vi "Status.vi"(8 "error in (no error)":errorcluster, 11 "Huber Settings":T1) -> (0 "error out":errorcluster, 1 "Connection Error":bool, 2 "Running":bool, 3 "Huber Settings":T1, 4 "Temp":i32)   [LabVIEW 2018, in "Huber Ministat 230 TCU.lvlib"]
uses:
  Huber Ministat 230 TCU.lvlib
  Huber Settings.ctl
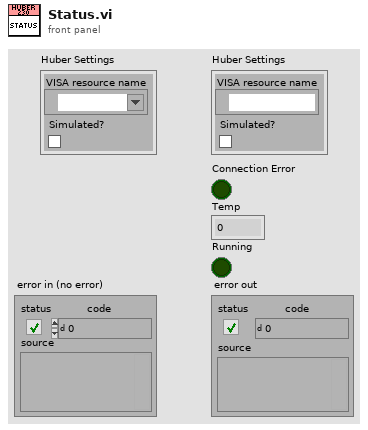
[diagram p1: front panel]
types:
  T1 = typedef "Huber Ministat 230 TCU.lvlib/Huber Settings.ctl" = cluster{"VISA resource name":refnum<visa-resource-name>, "Simulated?":bool}
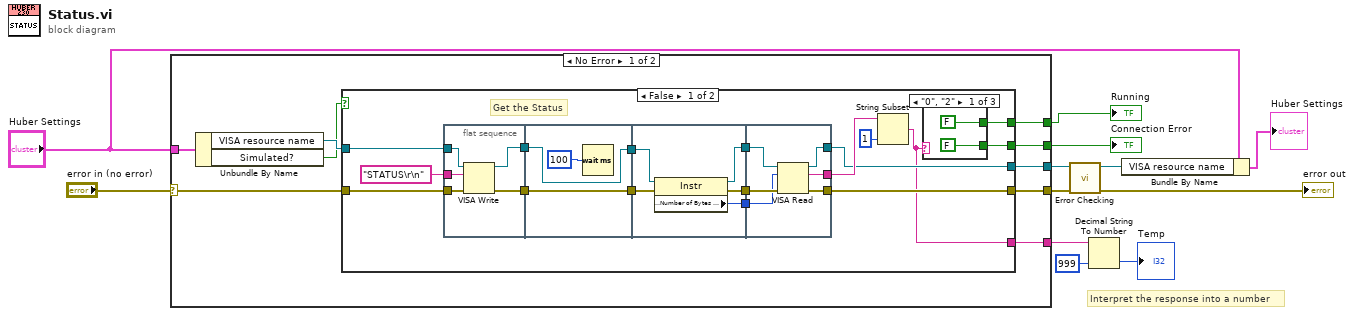
[diagram p0: block diagram]
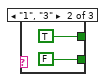
[diagram p2: hidden frame]
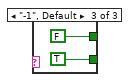
[diagram p3: hidden frame]
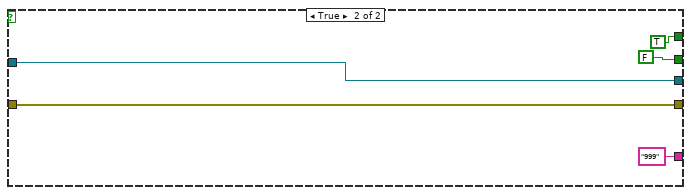
[diagram p4: hidden frame]
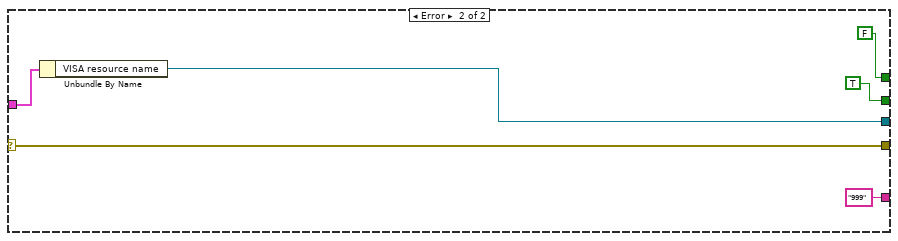
[diagram p5: hidden frame]
diagram:
  # "Interpret the response into a number"
  n1 = case shown="No Error" "error in (no error)" {
    selector: "error in (no error)" -> [w21 w74]
    tunnel: "Huber Settings" -> [w19 w73]
    tunnel: [w20 w74] -> w10
    tunnel: [w17 w72] -> w11
    tunnel: [w15 TRUE] -> w5
    tunnel: [w14 FALSE] -> w4
    tunnel: [w13 "999" ("read buffer")] -> w2
    frame No Error {
      n2 = Unbundle By Name(w19) -> ("VISA resource name"=w18:refnum<visa-resource-name>, "Simulated?"=w16:bool)
      n3 = case shown="False" w16 {
        tunnel: w21 -> [w24 w68]
        tunnel: [w26 w68] -> w20
        tunnel: [w27 w67] -> w17
        tunnel: w18 -> [w25 w67]
        tunnel: [w35 FALSE] -> w15
        tunnel: [w23 TRUE] -> w14
        tunnel: [w22 "999" ("read buffer")] -> w13
        frame False {
          # "Get the Status"
          n4 = flat-sequence {
            tunnel: "STATUS\r\n" ("string") -> [w49]
            tunnel: [w48] -> w37
            tunnel: [w47] -> w36
            tunnel: w25 -> [w46]
            tunnel: w24 -> [w45]
            tunnel: w37 -> [w51]
            tunnel: w36 -> [w50]
            tunnel: [w51] -> w29
            tunnel: [w50] -> w28
            tunnel: [w55] -> w32
            tunnel: [w54] -> w31
            tunnel: [w53] -> w30
            tunnel: w29 -> [w57]
            tunnel: w28 -> [w56]
            tunnel: [w63] -> w26
            tunnel: [w62] -> w33
            tunnel: [w61] -> w27
            tunnel: w32 -> [w60]
            tunnel: w31 -> [w59]
            tunnel: w30 -> [w58]
            frame #0 {
              n5 = VISA Write(VISA resource name=w46, write buffer=w49, error in (no error)=w45) -> (VISA resource name out=w48:refnum<visa-resource-name>, error out=w47:errorcluster)  [unwired: 1 out]
            }
            frame #1 {
              n6 = Wait (ms)(milliseconds to wait=u32 100) -> ()  [unwired: 1 out]
            }
            frame #2 {
              n7 = property class="Instr"(reference=w57, error in=w56) -> (reference out=w55:refnum<visa-resource-name>, error out=w54:errorcluster, "Serial Settings:Number of Bytes at Serial Port"=w53:u32)
            }
            frame #3 {
              n8 = VISA Read(VISA resource name=w60, byte count=w58, error in (no error)=w59) -> (VISA resource name out=w61:refnum<visa-resource-name>, read buffer=w62:string, error out=w63:errorcluster)  [unwired: 1 out]
            }
          }
          n9 = String Subset(string=w33, length (rest)=1 ("length (rest)")) -> (substring=w22:string)  [unwired: 1 in]
          n10 = case shown="\"0\", \"2\"" w22 {
            tunnel: [FALSE FALSE TRUE] -> w35
            tunnel: [FALSE TRUE FALSE] -> w23
            frame "0", "2" {
            }
            frame "1", "3" {
            }
            frame "-1", Default {
            }
          }
        }
        frame True {
        }
      }
    }
    frame Error {
      n11 = Unbundle By Name(w73) -> ("VISA resource name"=w72:refnum<visa-resource-name>)
    }
  }
  "Connection Error" <- w5
  "Running" <- w4
  n12 = call "Error Checking.vi"("error in (no error)"=w10, "VISA resource name"=w11) -> ("error out"=→"error out":errorcluster, "VISA resource name"=w8:refnum<visa-resource-name>)  [unwired: 7 in, 1 out]
  n13 = Decimal String To Number(string=w2, default (0L)=999 ("default (0 I32)")) -> (number=→"Temp":i32)  [unwired: 1 in, 1 out]
  n14 = Bundle By Name(cluster="Huber Settings", "VISA resource name"=w8) -> (→"Huber Settings":T1)
